vi "Get Control Default Value.vi"(8 "error in (no error)":errorcluster, 11 "Path":path) -> (0 "error out":errorcluster, 3 "Value":variant)   [LabVIEW 2015, in "Editor.lvclass"]
uses:
  Editor.lvclass
  <vilib>/Utility/error.llb/Error Cluster From Error Code.vi
  <vilib>/ErrorRing/Error Ring.xnode
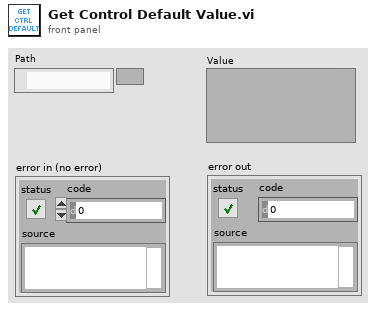
[diagram p1: front panel]
types:
  T1 = enum32{"invalid VI type", "Standard VI", "Control VI", "Global VI", "Polymorphic VI", "Configuration VI", "SubSystem", "Facade VI", "Method VI", "Statechart Diagram VI"}
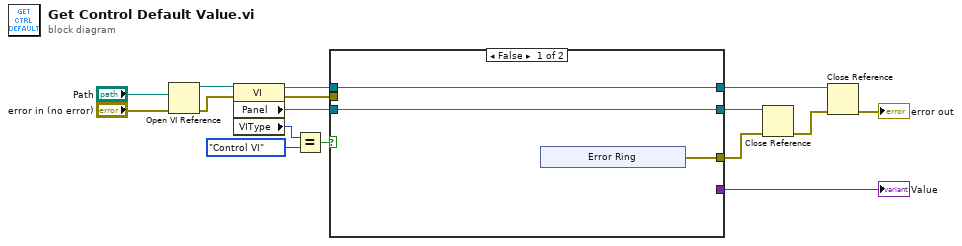
[diagram p0: block diagram]
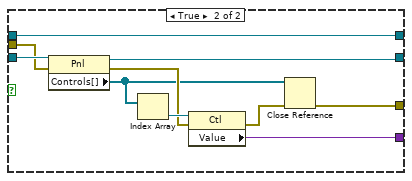
[diagram p2: hidden frame]
diagram:
  n1 = Open VI Reference(vi path="Path", error in (no error)="error in (no error)") -> (vi reference=w15:refnum<vi>, error out=w14:errorcluster)  [unwired: 4 in]
  n2 = property class="VI"(reference=w15, error in=w14) -> (reference out=w4:refnum<vi>, error out=w11:errorcluster, "Panel"=w13:refnum<vi>, "VIType"=w10:T1)
  n3 = Equal?(x=w10, y=T1."Control VI" ("VI Type")) -> (x = y?=w8:bool)
  n4 = case shown="False" w8 {
    tunnel: w13 -> [w19 w34]
    tunnel: w11 -> [_ w32]
    tunnel: [_ w28] -> w2
    tunnel: [w17 w27] -> w6
    tunnel: [w19 w26] -> w7
    tunnel: [w18 w25] -> w3
    tunnel: w4 -> [w18 w25]
    frame False {
      n5 = xnode "Error Ring"() -> ("error out"=w17:errorcluster)
    }
    frame True {
      n6 = property class="Pnl"(reference=w34, error in=w32) -> (reference out=w26:refnum<vi>, error out=w31:errorcluster, "Controls[]"=w30:refnum<vi>[])
      n7 = Index Array(array=w30) -> (element=w33:refnum<vi>)  [unwired: 1 in]
      n8 = property class="Ctl"(reference=w33, error in=w31) -> (error out=w29:errorcluster, "Value"=w28:variant)  [unwired: 1 out]
      n9 = Close Reference(reference=w30, error in (no error)=w29) -> (error out=w27:errorcluster)
    }
  }
  "Value" <- w2
  n10 = Close Reference(reference=w7, error in (no error)=w6) -> (error out=w5:errorcluster)
  n11 = Close Reference(reference=w3, error in (no error)=w5) -> (error out=→"error out":errorcluster)
